vi "Model Initial Values - Model Page.vi"(8 "error in (no error)":errorcluster, 11 "Node Ptr":T1 format="%.0x") -> (0 "error out":errorcluster)   [LabVIEW 2011, in "Model Initial Values Custom Device.lvlib"]
uses:
  Model Initial Values Custom Device.lvlib
  <vilib>/NI Veristand/Custom Device API/Custom Device Item Ref.ctl
  <vilib>/event_ctls.llb/eventvkey.ctl
  Model Initial Values - Global.vi
  <vilib>/NI Veristand/Custom Device API/Get Item Property (Double Array).vi
  <vilib>/NI Veristand/Custom Device API/Set Item Property (Double Array).vi
  <vilib>/NI Veristand/Custom Device API/Custom Device API.lvlib
panel:
  in  "Header":cluster{"Section Name":string}={"Section Name"="Model Inport Initial Values"}
  in  "Change Default":bool
  in  "Model Inports":i32(listbox)
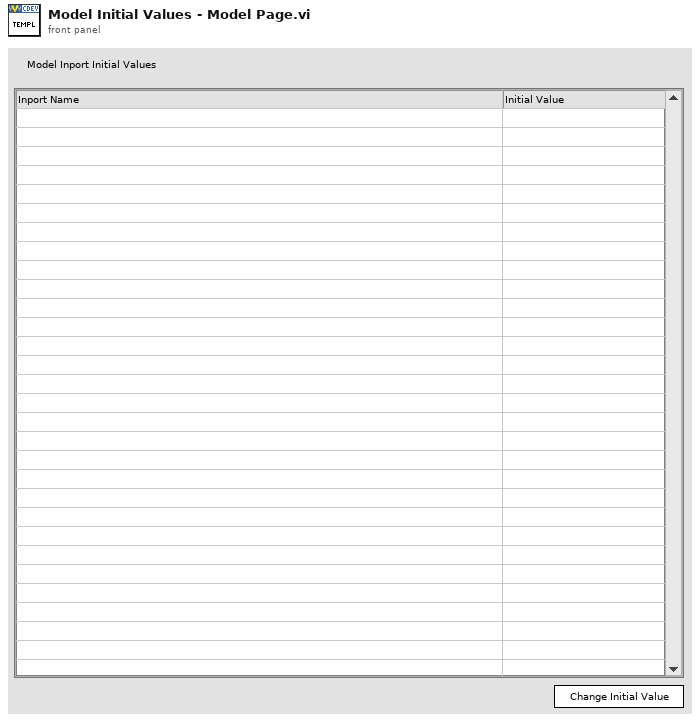
[diagram p1: front panel]
types:
  T1 = typedef "Custom Device API.lvlib/Custom Device Item Ref.ctl" = u64
  T2 = typedef "eventvkey.ctl" = enum16{"ASCII", "Enter", "Return", "Shift", "Ctrl", "Alt", "Cmd", "Opt", "Caps", "NumLock", "Clear", "Break", "Up", "Down", "Left", "Right", "Insert", "Delete", "Home", "End", "PageUp", "PageDown", "Escape", "Help", "Pause", "ScrollLock", "F1", "F2", "F3", "F4", "F5", "F6", "F7", "F8", "F9", "F10", "F11", "F12", "F13", "F14", "F15", "F16", "F17", "F18", "F19", "F20", "F21", "F22", "F23", "F24", "Play", "VolumeUp", "VolumeDown", "Mute", "Two Byte Char"}
  T3 = typedef "Custom Device API.lvlib/Custom Device Commands.ctl" = enum16{"Default", "Item renamed", "Shutdown", "Dynamic button pressed"}
  T4 = cluster{"Name":string, "Is Channel":bool, "GUID":string}
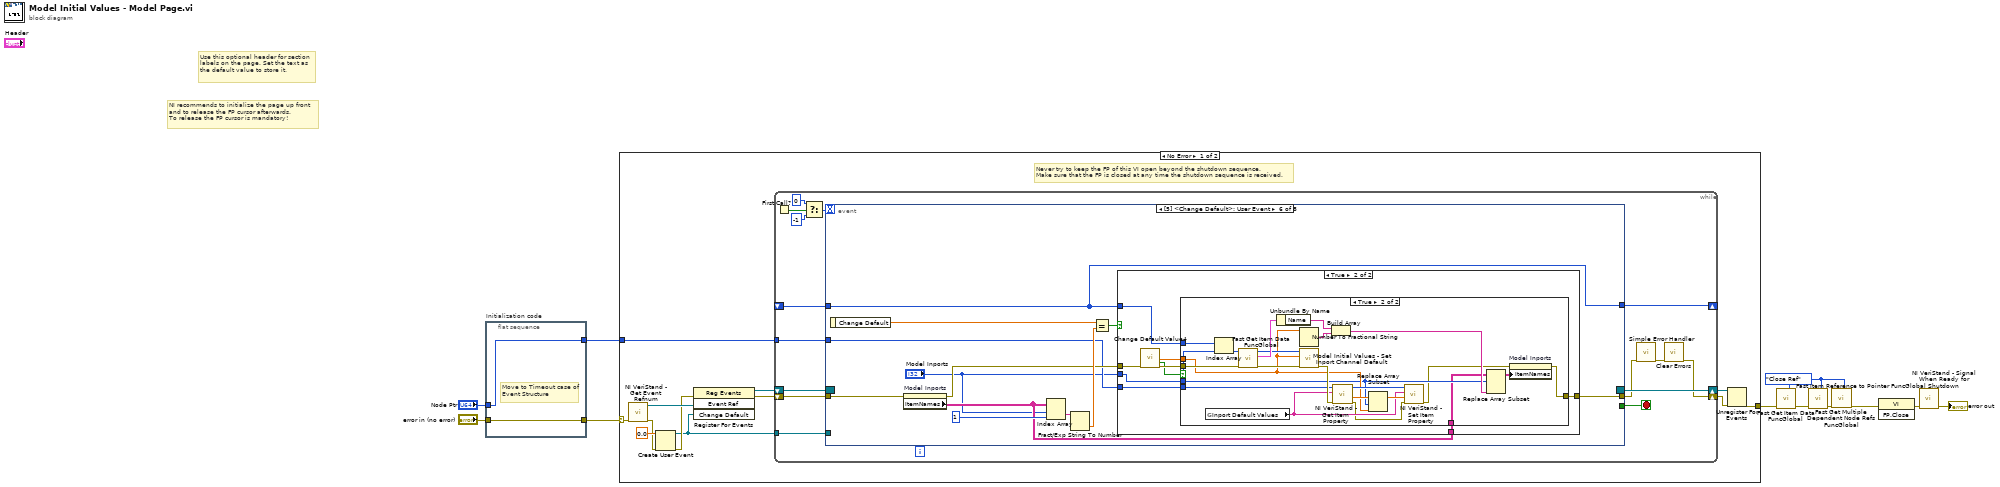
[diagram p0: block diagram]
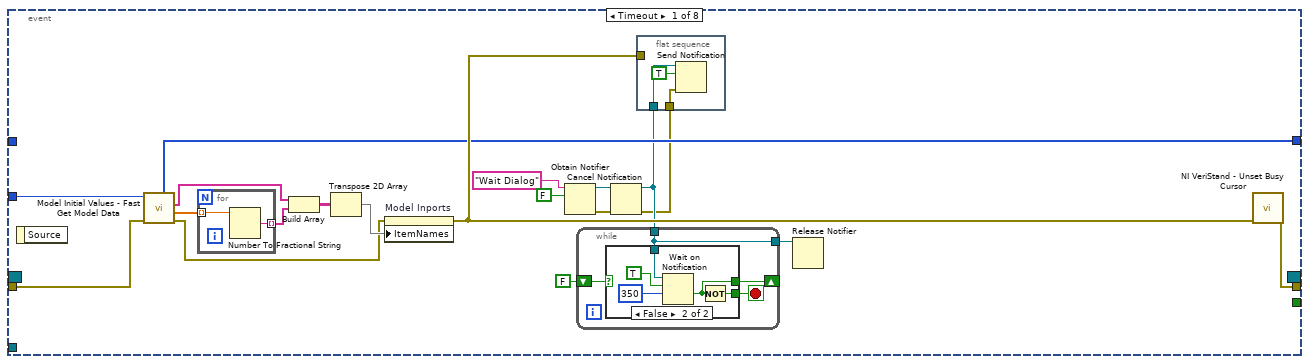
[diagram p2: hidden frame]
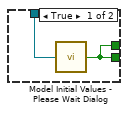
[diagram p3: hidden frame]
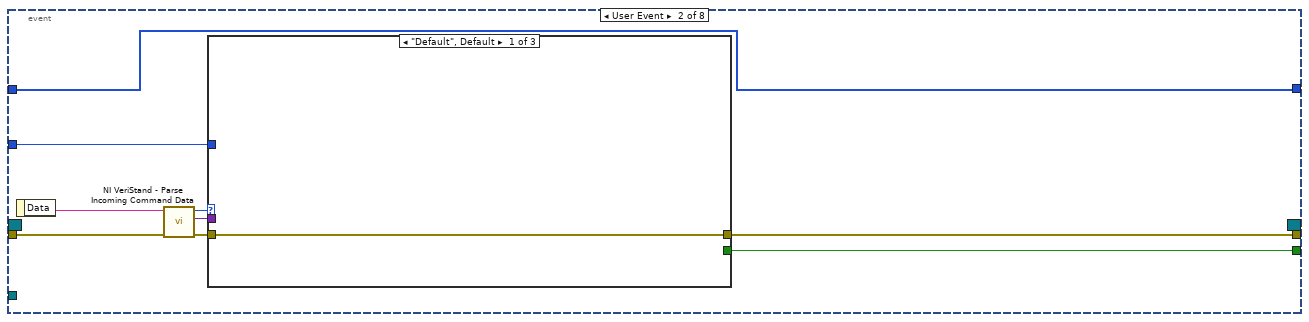
[diagram p4: hidden frame]
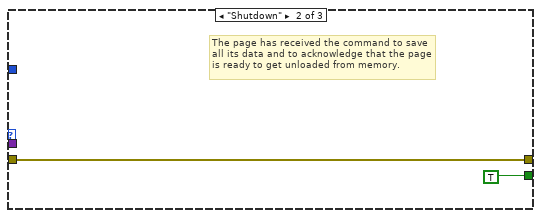
[diagram p5: hidden frame]
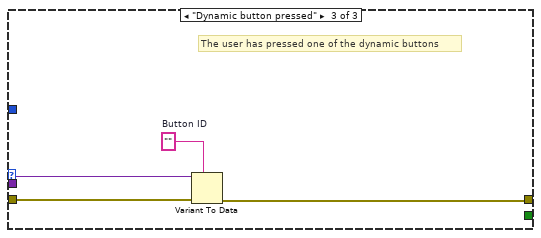
[diagram p6: hidden frame]
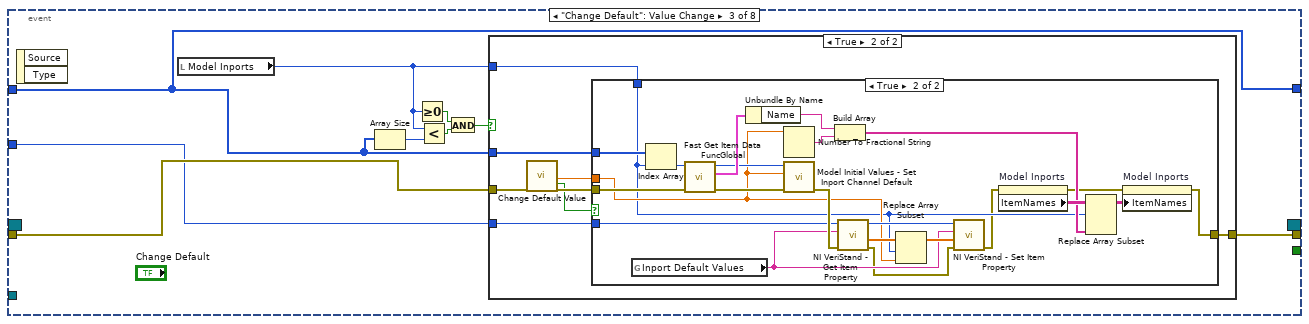
[diagram p7: hidden frame]
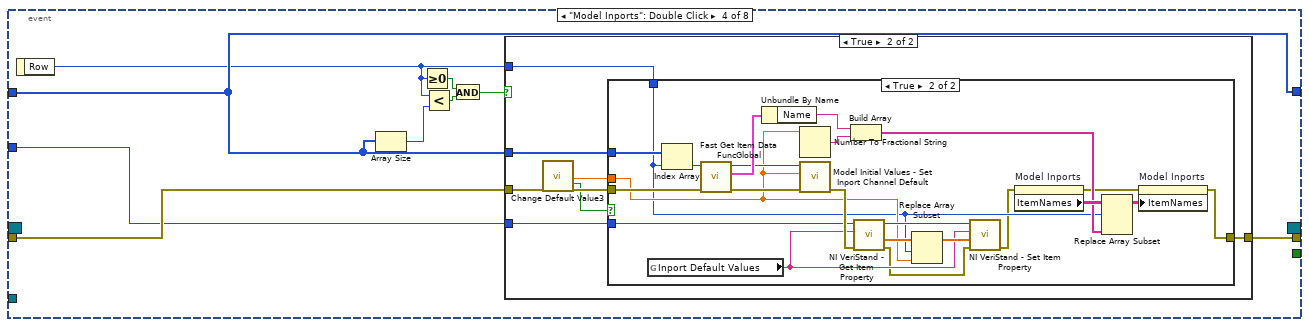
[diagram p10: hidden frame]
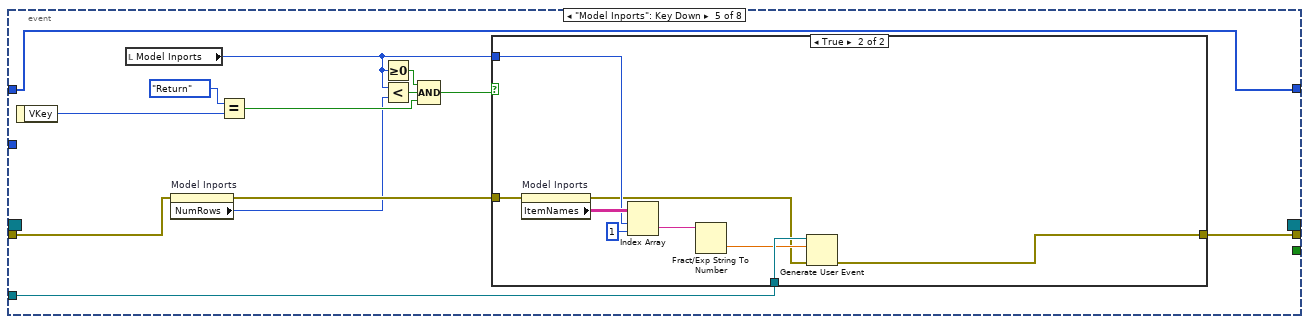
[diagram p13: hidden frame]
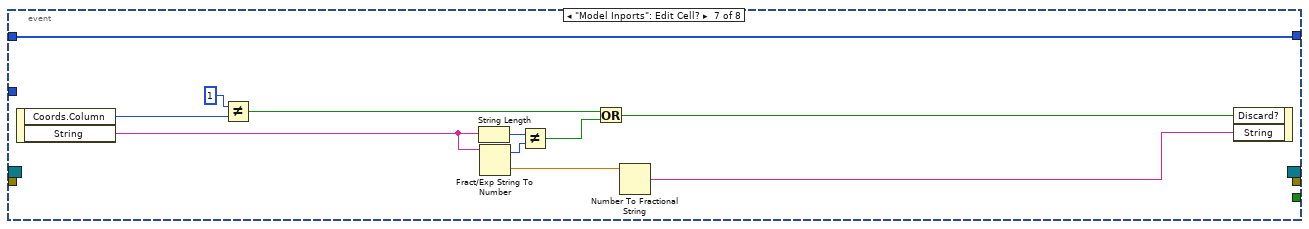
[diagram p17: hidden frame]
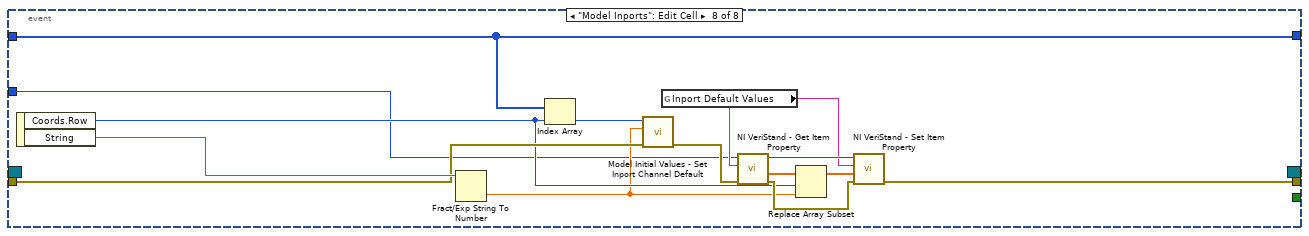
[diagram p18: hidden frame]
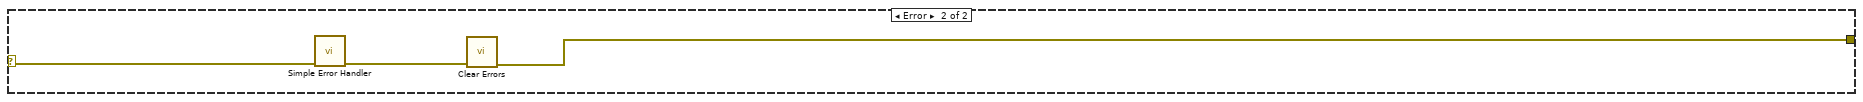
[diagram p19: hidden frame]
diagram:
  w2 = enum16{"Open or Add", "Close Ref"}."Close Ref" ("Action")
  # "Use this optional header for section labels on the page. Set the text as the default value to store it."
  # "NI recommends to initialize the page up front\nand to release the FP cursor afterwards.\nTo release the FP cursor is mandatory!"
  n1 = flat-sequence "Initialization code" {
    tunnel: "error in (no error)" -> [w13]
    tunnel: "Node Ptr" -> [w12]
    tunnel: [w13] -> w6
    tunnel: [w12] -> w7
    frame #0 {
      # "Move to Timeout case of Event Structure"
    }
  }
  n2 = case shown="No Error" w6 {
    selector: w6 -> [w18 w271]
    tunnel: [w23 w269] -> w5
    tunnel: w7 -> [w19 _]
    frame No Error {
      # "Never try to keep the FP of this VI open beyond the shutdown sequence.\nMake sure that the FP is closed at any time the shutdown sequence is received."
      n3 = call <vilib>:"NI VeriStand - Get Event Refnum.vi"("error in (no error)"=w18) -> ("error out"=w16:errorcluster, "Event Ref"=w22:refnum<user-event>)  [unwired: 9 out]
      n4 = Create User Event(user event datatype=0.0 ("Change Default"), error in=w16) -> (user event=w14:refnum<user-event>, error out=w15:errorcluster)
      n5 = register-events(error in=w15, w22, w14) -> (reference out=w20:refnum<event-registration>, error out=w21:errorcluster)  [unwired: 1 in]
      n6 = while {
        tunnel: w19 -> [w36]
        shift-right: [w33] -> w24
        shift-left: w21 -> [w39]
        shift-right: [w40] -> w25
        shift-left: w20 -> [w38]
        tunnel: w14 -> [w32]
        shift-right: [w27] -> _
        shift-left: _ -> [w26]
        stop <- w37 stop-if-true
        n7 = First Call?() -> (First Call?: T/F=w29:bool)
        n8 = Select(t=0, s=w29, f=-1) -> (s? t:f=w31:i32)
        n9 = event shown="[5] <Change Default>: User Event" {
          selector: w38 -> [_ _ _ _ _ _ _ _]
          dyn-events: [_ _ _ _ _ _ _ _] -> w40
          timeout: w31 -> [_ _ _ _ _ _ _ _]
          tunnel: w39 -> [w58 w84 w100 w136 w180 w209 _ w267]
          tunnel: [_ w80 _ _ _ _ _ _] -> w37
          tunnel: [w56 w79 w99 w134 w188 w205 _ w255] -> w35
          tunnel: w36 -> [w59 w78 w92 w135 _ w201 _ w256]
          tunnel: w32 -> [_ _ _ _ w177 _ _ _]
          tunnel: [w55 w76 w93 w139 w176 w200 w244 w259] -> w27
          tunnel: w26 -> [_ w76 w93 w139 w176 w200 w244 w259]
          event Timeout {
            n10 = event-data() -> ()  [unwired: 2 out]
            n11 = call "Model Initial Values - Fast Get Model Data.vi"("error in (no error)"=w58, "Local Model Ref in"=w59) -> ("error out"=w49:errorcluster, "Inport Default Values"=w51:dbl[], "Inport Names"=w52:string[], "Inport Refs"=w55:T1[])  [unwired: 4 in, 2 out]
            n12 = for {
              tunnel: w51 -> [w75] mode=indexing
              tunnel: [w74] -> w54 mode=indexing
              n13 = Number To Fractional String(number=w75) -> (F-format string=w74:string)  [unwired: 3 in]
            }
            n14 = Build Array(w52, w54) -> (w53:string[][])
            n15 = Transpose 2D Array(2D array=w53) -> (transposed array=w50:string[][])
            n16 = property on="Model Inports" class="MCListbox (strict)"(error in=w49, "ItemNames"=w50) -> (error out=w57:errorcluster)  [unwired: 1 in, 1 out]
            n17 = Obtain Notifier(name (unnamed)="Wait Dialog", notification data type=FALSE) -> (notifier out=w46:refnum<notifier>, error out=w43:errorcluster)  [unwired: 2 in, 1 out]
            n18 = Cancel Notification(0:w46, 3:w43) -> (8:w42:refnum<notifier>, 11:w41:errorcluster)  [unwired: 1 out]
            n19 = while {
              tunnel: w42 -> [w60]
              shift-right: [w61] -> _
              shift-left: FALSE -> [w62]
              tunnel: [w60] -> w44
              stop <- w63 stop-if-true
              n20 = case shown="False" w62 {
                tunnel: [w64 w68] -> w63
                tunnel: w60 -> [w65 w70]
                tunnel: [w64 w66] -> w61
                frame True {
                  n21 = call "Model Initial Values - Please Wait Dialog.vi"("notifier out"=w65) -> ("Boolean"=w64:bool)
                }
                frame False {
                  n22 = Wait on Notification(notifier=w70, ignore previous (F)=TRUE, timeout in ms (-1)=350) -> (timed out?=w66:bool)  [unwired: 1 in, 3 out]
                  n23 = Not(x=w66) -> (.not. x?=w68:bool)
                }
              }
            }
            n24 = flat-sequence {
              tunnel: w42 -> [w73]
              tunnel: w41 -> [w72]
              tunnel: w57 -> [_]
              frame #0 {
                n25 = Send Notification(notification=TRUE, notifier=w73, error in (no error)=w72) -> ()  [unwired: 2 out]
              }
            }
            n26 = Release Notifier(notifier=w44) -> ()  [unwired: 2 in, 3 out]
            n27 = call <vilib>:"NI VeriStand - Unset Busy Cursor.vi"("error in (no error)"=w57) -> ("error out"=w56:errorcluster)  [unwired: 10 out]
          }
          event User Event {
            n28 = event-data() -> ("Data"=w83:string)  [unwired: 1 out]
            n29 = call <vilib>:"NI VeriStand - Parse Incoming Command Data.vi"("error in (no error)"=w84, "Incoming data"=w83) -> ("error out"=w82:errorcluster, "Outgoing data"=w77:variant, "Action"=w81:T3)  [unwired: 7 out]
            n30 = case shown="\"Default\", Default" w81 {
              tunnel: w82 -> [w85 w86 w91]
              tunnel: [_ TRUE _] -> w80
              tunnel: [w85 w86 w88] -> w79
              tunnel: w78 -> [_ _ _]
              tunnel: w77 -> [_ _ w90]
              frame "Default", Default {
              }
              frame "Shutdown" {
                # "The page has received the command to save all its data and to acknowledge that the page is ready to get unloaded from memory."
              }
              frame "Dynamic button pressed" {
                w89 = ""  # Button ID
                # "The user has pressed one of the dynamic buttons"
                n31 = Variant To Data(error in=w91, type=w89, Variant=w90) -> (error out=w88:errorcluster)  [unwired: 1 out]
              }
            }
          }
          event "Change Default": Value Change {
            n32 = event-data() -> ()  [unwired: 3 out]
            n33 = local read "Model Inports"() -> (w95:i32)
            n34 = Array Size(array=w93) -> (size(s)=w98:i32)
            n35 = Greater Or Equal To 0?(x=w95) -> (x >= 0?=w97:bool)
            n36 = Less?(x=w95, y=w98) -> (x < y?=w96:bool)
            n37 = And(x=w97, y=w96) -> (x .and. y?=w94:bool)
            n38 = case shown="True" w94 {
              tunnel: w100 -> [w101 w106]
              tunnel: [w101 w109] -> w99
              tunnel: w93 -> [_ w108]
              tunnel: w95 -> [_ w107]
              tunnel: w92 -> [_ w102]
              frame False {
              }
              frame True {
                n39 = call "Change Default Value"("error in (no error)"=w106) -> ("Default Value"=w104:dbl, "OK"=w103:bool, "error out"=w105:errorcluster)  [unwired: 16 in]
                n40 = case shown="True" w103 {
                  tunnel: [w110 w127] -> w109
                  tunnel: w108 -> [_ w126]
                  tunnel: w107 -> [_ w112]
                  tunnel: w105 -> [w110 w123]
                  tunnel: w104 -> [_ w113]
                  tunnel: w102 -> [_ w119]
                  frame False {
                  }
                  frame True {
                    n41 = global read "Model Initial Values - Global.vi" "Inport Default Values"() -> (w116:string)
                    n42 = Index Array(array=w126, index=w112) -> (element=w125:T1)
                    n43 = call "Fast Get Item Data FuncGlobal.vi"("error in (no error)"=w123, "Item Ref in"=w125) -> ("error out"=w122:errorcluster, "Item Info"=w124:T4, "Item Ref out"=w121:T1)  [unwired: 6 in, 1 out]
                    n44 = Unbundle By Name(w124) -> ("Name"=w131:string)
                    n45 = Number To Fractional String(number=w113) -> (F-format string=w132:string)  [unwired: 3 in]
                    n46 = call "Model Initial Values - Set Inport Channel Default.vi"("error in"=w122, "Default Value"=w113, "Item Ref in"=w121) -> ("error out"=w120:errorcluster)  [unwired: 7 in, 1 out]
                    n47 = Build Array(w131, w132) -> (w130:string[])
                    n48 = call-poly <vilib>:"NI VeriStand - Get Item Property.vi"("error in (no error)"=w120, "Property Name"=w116, "Item Ref in"=w119) -> ("error out"=w114:errorcluster, "Value"=w118:dbl[], "Item Ref out"=w115:T1)  [unwired: 5 in, 1 out]
                    n49 = Replace Array Subset(array=w118, new element=w113, index=w112) -> (w117:dbl[])
                    n50 = call-poly <vilib>:"NI VeriStand - Set Item Property.vi"("error in (no error)"=w114, "Value"=w117, "Property Name"=w116, "Item Ref in"=w115) -> ("error out"=w111:errorcluster)  [unwired: 5 in, 2 out]
                    n51 = property on="Model Inports" class="MCListbox (strict)"(error in=w111) -> (error out=w128:errorcluster, "ItemNames"=w133:string[][])  [unwired: 1 in, 1 out]
                    n52 = Replace Array Subset(array=w133, new element=w130, index (row)=w112) -> (w129:string[][])  [unwired: 1 in]
                    n53 = property on="Model Inports" class="MCListbox (strict)"(error in=w128, "ItemNames"=w129) -> (error out=w127:errorcluster)  [unwired: 1 in, 1 out]
                  }
                }
              }
            }
          }
          event "Model Inports": Double Click {
            n54 = event-data() -> ("Row"=w138:i32)  [unwired: 1 out]
            n55 = Array Size(array=w139) -> (size(s)=w142:i32)
            n56 = Greater Or Equal To 0?(x=w138) -> (x >= 0?=w141:bool)
            n57 = Less?(x=w138, y=w142) -> (x < y?=w140:bool)
            n58 = And(x=w141, y=w140) -> (x .and. y?=w137:bool)
            n59 = case shown="True" w137 {
              tunnel: w136 -> [w143 w148]
              tunnel: [w143 w151] -> w134
              tunnel: w139 -> [_ w150]
              tunnel: w138 -> [_ w149]
              tunnel: w135 -> [_ w144]
              frame False {
              }
              frame True {
                n60 = call "Change Default Value3"("error in (no error)"=w148) -> ("Default Value"=w146:dbl, "OK"=w145:bool, "error out"=w147:errorcluster)  [unwired: 16 in]
                n61 = case shown="True" w145 {
                  tunnel: [w152 w169] -> w151
                  tunnel: w150 -> [_ w168]
                  tunnel: w149 -> [_ w154]
                  tunnel: w147 -> [w152 w165]
                  tunnel: w146 -> [_ w155]
                  tunnel: w144 -> [_ w161]
                  frame False {
                  }
                  frame True {
                    n62 = global read "Model Initial Values - Global.vi" "Inport Default Values"() -> (w158:string)
                    n63 = Index Array(array=w168, index=w154) -> (element=w167:T1)
                    n64 = call "Fast Get Item Data FuncGlobal.vi"("error in (no error)"=w165, "Item Ref in"=w167) -> ("error out"=w164:errorcluster, "Item Info"=w166:T4, "Item Ref out"=w163:T1)  [unwired: 6 in, 1 out]
                    n65 = Unbundle By Name(w166) -> ("Name"=w173:string)
                    n66 = Number To Fractional String(number=w155) -> (F-format string=w174:string)  [unwired: 3 in]
                    n67 = call "Model Initial Values - Set Inport Channel Default.vi"("error in"=w164, "Default Value"=w155, "Item Ref in"=w163) -> ("error out"=w162:errorcluster)  [unwired: 7 in, 1 out]
                    n68 = Build Array(w173, w174) -> (w172:string[])
                    n69 = call-poly <vilib>:"NI VeriStand - Get Item Property.vi"("error in (no error)"=w162, "Property Name"=w158, "Item Ref in"=w161) -> ("error out"=w156:errorcluster, "Value"=w160:dbl[], "Item Ref out"=w157:T1)  [unwired: 5 in, 1 out]
                    n70 = Replace Array Subset(array=w160, new element=w155, index=w154) -> (w159:dbl[])
                    n71 = call-poly <vilib>:"NI VeriStand - Set Item Property.vi"("error in (no error)"=w156, "Value"=w159, "Property Name"=w158, "Item Ref in"=w157) -> ("error out"=w153:errorcluster)  [unwired: 5 in, 2 out]
                    n72 = property on="Model Inports" class="MCListbox (strict)"(error in=w153) -> (error out=w170:errorcluster, "ItemNames"=w175:string[][])  [unwired: 1 in, 1 out]
                    n73 = Replace Array Subset(array=w175, new element=w172, index (row)=w154) -> (w171:string[][])  [unwired: 1 in]
                    n74 = property on="Model Inports" class="MCListbox (strict)"(error in=w170, "ItemNames"=w171) -> (error out=w169:errorcluster)  [unwired: 1 in, 1 out]
                  }
                }
              }
            }
          }
          event "Model Inports": Key Down {
            n75 = event-data() -> ("VKey"=w181:T2)  [unwired: 1 out]
            n76 = local read "Model Inports"() -> (w185:i32)
            n77 = property on="Model Inports" class="MCListbox (strict)"(error in=w180) -> (error out=w179:errorcluster, "NumRows"=w178:u32)  [unwired: 1 in, 1 out]
            n78 = Equal?(x=eventvkey."Return" ("y"), y=w181) -> (x = y?=w183:bool)
            n79 = Greater Or Equal To 0?(x=w185) -> (x >= 0?=w187:bool)
            n80 = Less?(x=w185, y=w178) -> (x < y?=w186:bool)
            n81 = Compound Arithmetic op=AND(w187, w186, w183) -> (w184:bool)
            n82 = case shown="True" w184 {
              tunnel: w179 -> [w189 w198]
              tunnel: [w189 w190] -> w188
              tunnel: w185 -> [_ w196]
              tunnel: w177 -> [_ w193]
              frame False {
              }
              frame True {
                n83 = property on="Model Inports" class="MCListbox (strict)"(error in=w198) -> (error out=w191:errorcluster, "ItemNames"=w197:string[][])  [unwired: 1 in, 1 out]
                n84 = Index Array(array=w197, index (row)=w196, index (col)=1 ("disabled index (col)")) -> (element=w194:string)
                n85 = Fract/Exp String To Number(string=w194) -> (number=w192:dbl)  [unwired: 3 in, 1 out]
                n86 = Generate User Event(user event=w193, event data cluster=w192, error in=w191) -> (error out=w190:errorcluster)  [unwired: 1 out]
              }
            }
          }
          event User Event {
            n87 = event-data() -> ("Change Default"=w207:dbl)  [unwired: 1 out]
            n88 = property on="Model Inports" class="MCListbox (strict)"(error in=w209) -> (error out=w203:errorcluster, "ItemNames"=w202:string[][])  [unwired: 1 in, 1 out]
            n89 = Index Array(array=w202, index (row)="Model Inports", index (col)=1 ("disabled index (col)")) -> (element=w208:string)
            n90 = Fract/Exp String To Number(string=w208) -> (number=w206:dbl)  [unwired: 3 in, 1 out]
            n91 = Equal?(x=w207, y=w206) -> (x = y?=w204:bool)
            n92 = case shown="True" w204 {
              tunnel: w203 -> [w211 w217]
              tunnel: [w211 w220] -> w205
              tunnel: w200 -> [_ w219]
              tunnel: "Model Inports" -> [_ w218]
              tunnel: w201 -> [_ w213]
              tunnel: w202 -> [_ w212]
              frame False {
              }
              frame True {
                n93 = call "Change Default Value4"("error in (no error)"=w217) -> ("Default Value"=w215:dbl, "OK"=w214:bool, "error out"=w216:errorcluster)  [unwired: 16 in]
                n94 = case shown="True" w214 {
                  tunnel: [w221 w239] -> w220
                  tunnel: w219 -> [_ w238]
                  tunnel: w218 -> [_ w224]
                  tunnel: w216 -> [w221 w235]
                  tunnel: w215 -> [_ w225]
                  tunnel: w213 -> [_ w231]
                  tunnel: w212 -> [_ w223]
                  frame False {
                  }
                  frame True {
                    n95 = global read "Model Initial Values - Global.vi" "Inport Default Values"() -> (w228:string)
                    n96 = Index Array(array=w238, index=w224) -> (element=w237:T1)
                    n97 = call "Fast Get Item Data FuncGlobal.vi"("error in (no error)"=w235, "Item Ref in"=w237) -> ("error out"=w234:errorcluster, "Item Info"=w236:T4, "Item Ref out"=w233:T1)  [unwired: 6 in, 1 out]
                    n98 = Unbundle By Name(w236) -> ("Name"=w242:string)
                    n99 = Number To Fractional String(number=w225) -> (F-format string=w243:string)  [unwired: 3 in]
                    n100 = call "Model Initial Values - Set Inport Channel Default.vi"("error in"=w234, "Default Value"=w225, "Item Ref in"=w233) -> ("error out"=w232:errorcluster)  [unwired: 7 in, 1 out]
                    n101 = Build Array(w242, w243) -> (w241:string[])
                    n102 = call-poly <vilib>:"NI VeriStand - Get Item Property.vi"("error in (no error)"=w232, "Property Name"=w228, "Item Ref in"=w231) -> ("error out"=w226:errorcluster, "Value"=w230:dbl[], "Item Ref out"=w227:T1)  [unwired: 5 in, 1 out]
                    n103 = Replace Array Subset(array=w230, new element=w225, index=w224) -> (w229:dbl[])
                    n104 = call-poly <vilib>:"NI VeriStand - Set Item Property.vi"("error in (no error)"=w226, "Value"=w229, "Property Name"=w228, "Item Ref in"=w227) -> ("error out"=w222:errorcluster)  [unwired: 5 in, 2 out]
                    n105 = Replace Array Subset(array=w223, new element=w241, index (row)=w224) -> (w240:string[][])  [unwired: 1 in]
                    n106 = property on="Model Inports" class="MCListbox (strict)"(error in=w222, "ItemNames"=w240) -> (error out=w239:errorcluster)  [unwired: 1 in, 1 out]
                  }
                }
              }
            }
          }
          event "Model Inports": Edit Cell? {
            n107 = event-data() -> ("Coords.Column"=w254:i32, "String"=w252:string)  [unwired: 1 out]
            n108 = Not Equal?(x=1 ("y"), y=w254) -> (x != y?=w251:bool)
            n109 = String Length(string=w252) -> (length=w250:i32)
            n110 = Fract/Exp String To Number(string=w252) -> (offset past number=w249:i32, number=w246:dbl)  [unwired: 3 in]
            n111 = Not Equal?(x=w250, y=w249) -> (x != y?=w247:bool)
            n112 = Or(x=w251, y=w247) -> (x .or. y?=w248:bool)
            n113 = Number To Fractional String(number=w246) -> (F-format string=w245:string)  [unwired: 3 in]
            n114 = event-data("Discard?"=w248, "String"=w245) -> ()  [unwired: 1 in, 1 out]
          }
          event "Model Inports": Edit Cell {
            n115 = event-data() -> ("Coords.Row"=w258:i32, "String"=w268:string)  [unwired: 1 out]
            n116 = Fract/Exp String To Number(string=w268) -> (number=w257:dbl)  [unwired: 3 in, 1 out]
            n117 = Index Array(array=w259, index=w258) -> (element=w266:T1)
            n118 = call "Model Initial Values - Set Inport Channel Default.vi"("error in"=w267, "Default Value"=w257, "Item Ref in"=w266) -> ("error out"=w260:errorcluster)  [unwired: 7 in, 1 out]
            n119 = global read "Model Initial Values - Global.vi" "Inport Default Values"() -> (w263:string)
            n120 = call-poly <vilib>:"NI VeriStand - Get Item Property.vi"("error in (no error)"=w260, "Property Name"=w263, "Item Ref in"=w256) -> ("error out"=w265:errorcluster, "Value"=w261:dbl[], "Item Ref out"=w264:T1)  [unwired: 5 in, 1 out]
            n121 = Replace Array Subset(array=w261, new element=w257, index=w258) -> (w262:dbl[])
            n122 = call-poly <vilib>:"NI VeriStand - Set Item Property.vi"("error in (no error)"=w265, "Value"=w262, "Property Name"=w263, "Item Ref in"=w264) -> ("error out"=w255:errorcluster)  [unwired: 5 in, 2 out]
          }
        }
        n123 = call <vilib>:"Simple Error Handler.vi"("error in (no error)"=w35) -> ("error out"=w34:errorcluster)  [unwired: 1 in, 7 out]
        n124 = call <vilib>:"Clear Errors.vi"("error in (no error)"=w34) -> ("error out"=w33:errorcluster)  [unwired: 6 out]
      }
      n125 = Unregister For Events(event registration refnum=w25, error in=w24) -> (error out=w23:errorcluster)
    }
    frame Error {
      n126 = call <vilib>:"Simple Error Handler.vi"("error in (no error)"=w271) -> ("error out"=w270:errorcluster)  [unwired: 1 in, 7 out]
      n127 = call <vilib>:"Clear Errors.vi"("error in (no error)"=w270) -> ("error out"=w269:errorcluster)  [unwired: 6 out]
    }
  }
  n128 = call "Fast Get Item Data FuncGlobal.vi"("Action"=w2, "error in (no error)"=w5) -> ("error out"=w4:errorcluster)  [unwired: 6 in, 3 out]
  n129 = call "Fast Item Reference to Pointer FuncGlobal.vi"("Action"=w2, "error in (no error)"=w4) -> ("error out"=w3:errorcluster)  [unwired: 6 in, 3 out]
  n130 = call "Fast Get Multiple Dependent Node Refs FuncGlobal.vi"("Action"=w2, "error in (no error)"=w3) -> ("error out"=w1:errorcluster)  [unwired: 7 in, 2 out]
  n131 = invoke class="VI" method="FP.Close"(error in=w1) -> (error out=w11:errorcluster)  [unwired: 2 in, 2 out]
  n132 = call <vilib>:"NI VeriStand - Signal When Ready for Shutdown.vi"("error in (no error)"=w11) -> ("error out"=→"error out":errorcluster)  [unwired: 10 out]
